vi "signal.vi"(1 "Parametros Actuales IN":T1, 2 "Sound Parameters":cluster{"# samples":u32, "tiempos (ms)":dbl}, 3 "Señal de Control IN":dbl[](array[numeric])) -> (0 "Out":dbl[](array[numeric]))   [LabVIEW 2010]
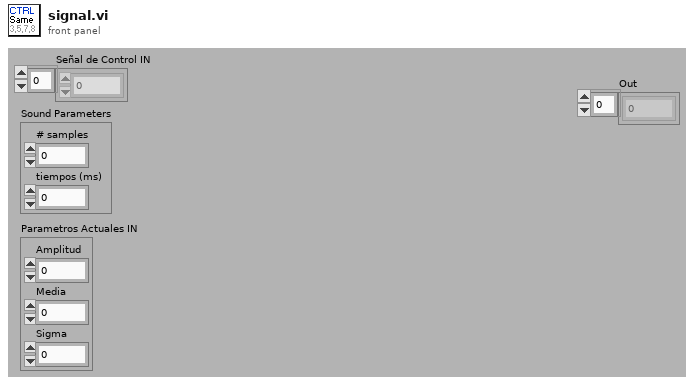
[diagram p1: front panel]
types:
  T1 = cluster{"Amplitud":dbl, "Media":dbl, "Sigma":dbl}
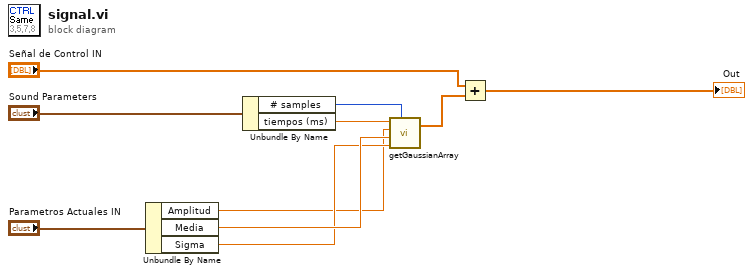
[diagram p0: block diagram]
diagram:
  n1 = Unbundle By Name("Parametros Actuales IN") -> ("Amplitud"=w1:dbl, "Media"=w3:dbl, "Sigma"=w2:dbl)
  n2 = Unbundle By Name("Sound Parameters") -> ("# samples"=w6:u32, "tiempos (ms)"=w5:dbl)
  n3 = call "getGaussianArray.vi"("tiempo (ms)"=w5, "Amplitud"=w1, "t0 (ms)"=w3, "Sigma (ms)"=w2, "#samples"=w6) -> ("Y out"=w9:dbl[])  [unwired: 1 out]
  n4 = Add(x="Señal de Control IN", y=w9) -> (x+y=→"Out":dbl[])
